vi "Open Interface.vi"(6 "read_timeout (1000)":i32=1000, 8 "error in (no error)":errorcluster, 9 "capture_size (65536)":i32=65536, 10 "promiscuous mode (T)":bool=TRUE, 11 "adapter (0)":i32) -> (0 "error out":errorcluster, 3 "pcap reference":u32)   [LabVIEW 2017, in "lvwpcap.lvlib"]
uses:
  lvwpcap.lvlib
  LVpcap.dll
panel:
  in  "pcap (dummy)":u32
  # "Select Help»Show Context Help and move the cursor over the VI icon to display help for this VI."
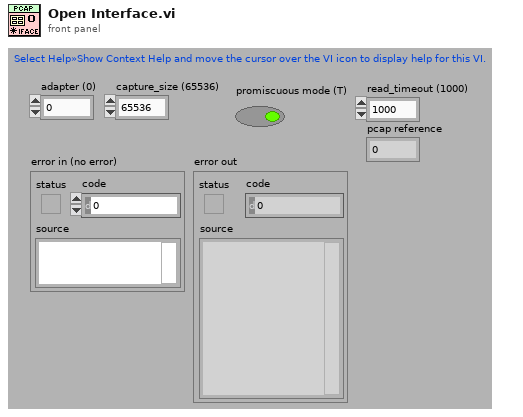
[diagram p1: front panel]
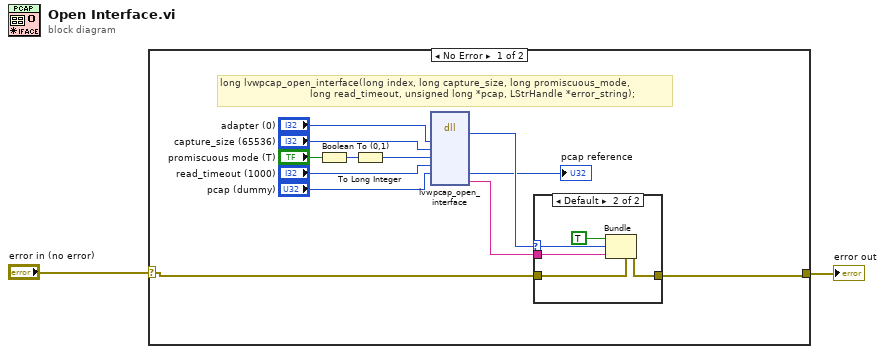
[diagram p0: block diagram]
diagram:
  n1 = case shown="No Error" "error in (no error)" {
    selector: "error in (no error)" -> [w4 w21]
    tunnel: [w3 w21] -> w1
    frame No Error {
      # "long lvwpcap_open_interface(long index, long capture_size, long promiscuous_mode,\n                              long read_timeout, unsigned long *pcap, LStrHandle *error_string);"
      n2 = Boolean To (0,1)(Boolean="promiscuous mode (T)") -> (0, 1=w9:i16)
      n3 = To Long Integer(number=w9) -> (32bit integer=w8:i32)
      n4 = dll-call lib="C:/Users/Michaello/Desktop/MGR NOWEEEEEEEEEEEEEE/MR PROFINET 2017/Lib/WinPcap/LVpcap.dll" fn="lvwpcap_open_interface"("index"="adapter (0)", "capture_size"="capture_size (65536)", "promiscuous_mode"=w8, "read_timeout"="read_timeout (1000)", "pcap"="pcap (dummy)") -> ("return type"=w13:i32, "pcap"=→"pcap reference":u32, "error_string"=w12:string)  [unwired: 8 in, 2 out]
      n5 = case shown="Default" w13 {
        selector: w13 -> [_ w19]
        tunnel: w12 -> [_ w18]
        tunnel: w4 -> [w15 w20]
        tunnel: [w15 w16] -> w3
        frame 0 {
        }
        frame Default {
          n6 = Bundle(cluster=w20, "status"=TRUE, "code"=w19, "source"=w18) -> (w16:errorcluster)
        }
      }
    }
    frame Error {
    }
  }
  "error out" <- w1
